vi "CAENHV Get Bd Param Info.vi"(8 "error in (no error)":errorcluster, 10 "slot":u16, 11 "handle":i32) -> (0 "error out":errorcluster, 3 "ParNameList":string[](array[string]))   [LabVIEW 2009, in "CAENHVWrapper.lvlib"]
doc: "CAENHVLIB_API CAENHVRESULT CAENHV_GetBdParamInfo(int handle, \n ushort slot, char **ParNameList);"
uses:
  <userlib>/CAENHVWrapper/CAENHVWrapper.lvlib
  <vilib>/Utility/importsl/GetValueByPointer/GetValueByPointer.xnode
  <vilib>/Utility/importsl/GetValueByPointer/datatype.ctl
  <userlib>/CAENHVWrapper/CAENHVWrapper.dll
  resource/lvimptsl.dll
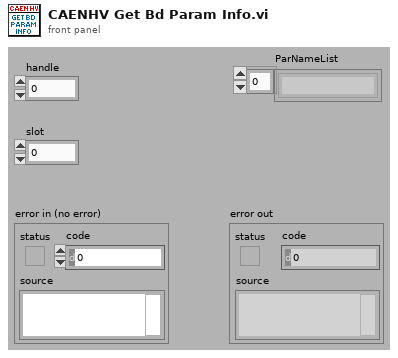
[diagram p1: front panel]
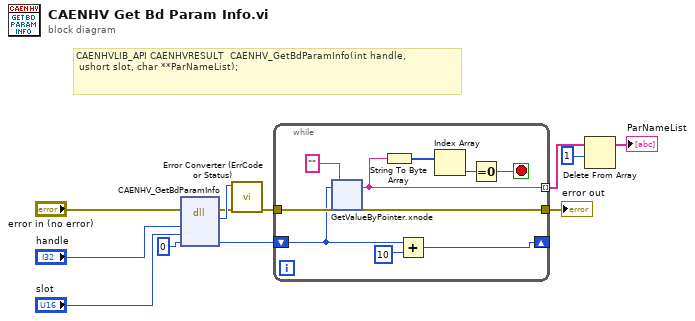
[diagram p0: block diagram]
diagram:
  # "CAENHVLIB_API CAENHVRESULT  CAENHV_GetBdParamInfo(int handle, \n ushort slot, char **ParNameList);"
  n1 = dll-call lib="C:/Program Files/National Instruments/LabVIEW 2009/user.lib/CAENHVWrapper/CAENHVWrapper.*" fn="CAENHV_GetBdParamInfo"(error in="error in (no error)", "handle"="handle", "slot"="slot", "ParNameList"=i64 0) -> (error out=w8:errorcluster, "return type"=w9:i32, "ParNameList"=w5:i64)  [unwired: 4 in, 1 out]
  n2 = call <userlib>:"Error Converter (ErrCode or Status).vi"("error in (no error)"=w8, "error code"=w9) -> ("error out"=w4:errorcluster)  [unwired: 9 in]
  n3 = while {
    shift-right: [w18] -> _
    shift-left: w5 -> [w20]
    tunnel: w4 -> [w22]
    tunnel: [w21] -> w6
    tunnel: [w16] -> w3 mode=indexing
    stop <- w15 stop-if-true
    n4 = xnode "GetValueByPointer.xnode"("Pointer"=w20, "InputType"="", "ErrorIn"=w22) -> ("Output"=w16:string, "ErrorOut"=w21:errorcluster)  [unwired: 1 in]
    n5 = String To Byte Array(string=w16) -> (unsigned byte array=w14:u8[])
    n6 = Add(x=w20, y=i64 10) -> (x+y=w18:i64)
    n7 = Index Array(array=w14) -> (element=w13:u8)  [unwired: 1 in]
    n8 = Equal To 0?(x=w13) -> (x = 0?=w15:bool)
  }
  "error out" <- w6
  n9 = Delete From Array(array=w3, length=1) -> (array with subset deleted=→"ParNameList":string[])  [unwired: 1 in, 1 out]
